vi "TPP-printer-v3.vi"() -> ()   [LabVIEW 2015]
uses:
  <vilib>/DAQmx/write.llb/DAQmx Write (Digital Bool 1Line 1Point).vi
  <vilib>/Utility/file.llb/Read Delimited Spreadsheet (I64).vi
  <vilib>/DAQmx/create/channels.llb/DAQmx Create Channel (DO-Digital Output).vi
  <vilib>/DAQmx/miscellaneous.llb/DAQmx Fill In Error Info.vi
  <vilib>/Platform/NI_3dgraph.lvlib
  Kinesis/Thorlabs.MotionControl.Controls.dll
panel:
  in  "f_objecitve(mm)":dbl=1.8
  in  "f_tubelens(mm)":dbl=200.0
  in  "f_scanlens(mm)":dbl=50.0
  out "%":dbl=1.1971958040155672 format="%#.2g"
  in  "读取点阵文件":path=path "C:/Users/Hongq/Desktop/grating.txt"
  in  "停止":bool
  out "每层耗时/s":dbl format="%#.2g"
  out "每行耗时/s":dbl=0.4888782501220703 format="%#.2g"
  out "每点耗时/ms":dbl=4.009246826171875 format="%#.0g"
  out "当前完成量：":u8(slide)=1 scale=0.0..100.0
  out "耗时/min":dbl=0.11883490880330404 format="%#.2g"
  out "模型XYZ坐标表":dbl[][](array[numeric])
  in  "模型高/um":dbl=1.0
  in  "总体预览":refnum<k7>(container)
  in  "刷新预览":bool
  in  "Z轴驱动序列号":string="27000001"
  in  "KCubeDCServoControl":refnum<k24>(container)
  in  "XY速度(um/s)":dbl
  out "XYZ当前坐标/um":dbl[](array[numeric])=[-0.4166666666666667, -0.1875, 0.0, 7.132113933563232, 7.091063499450684, 0.0] format="%#.2g"
  in  "比例因子(V/°)":dbl=0.5
  in  "AO通道：X前Y后":tag="Dev1/ao0:1"
  out "当前扫描速度(um/s)":dbl
  in  "DO通道：shutter控制":tag="Dev1/port1/line0" caption="线"
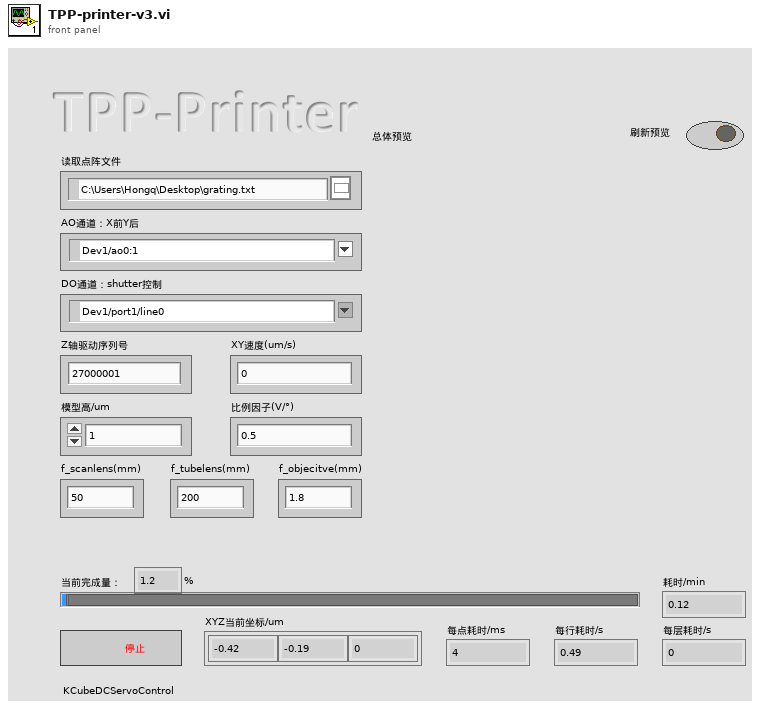
[diagram p1: front panel]
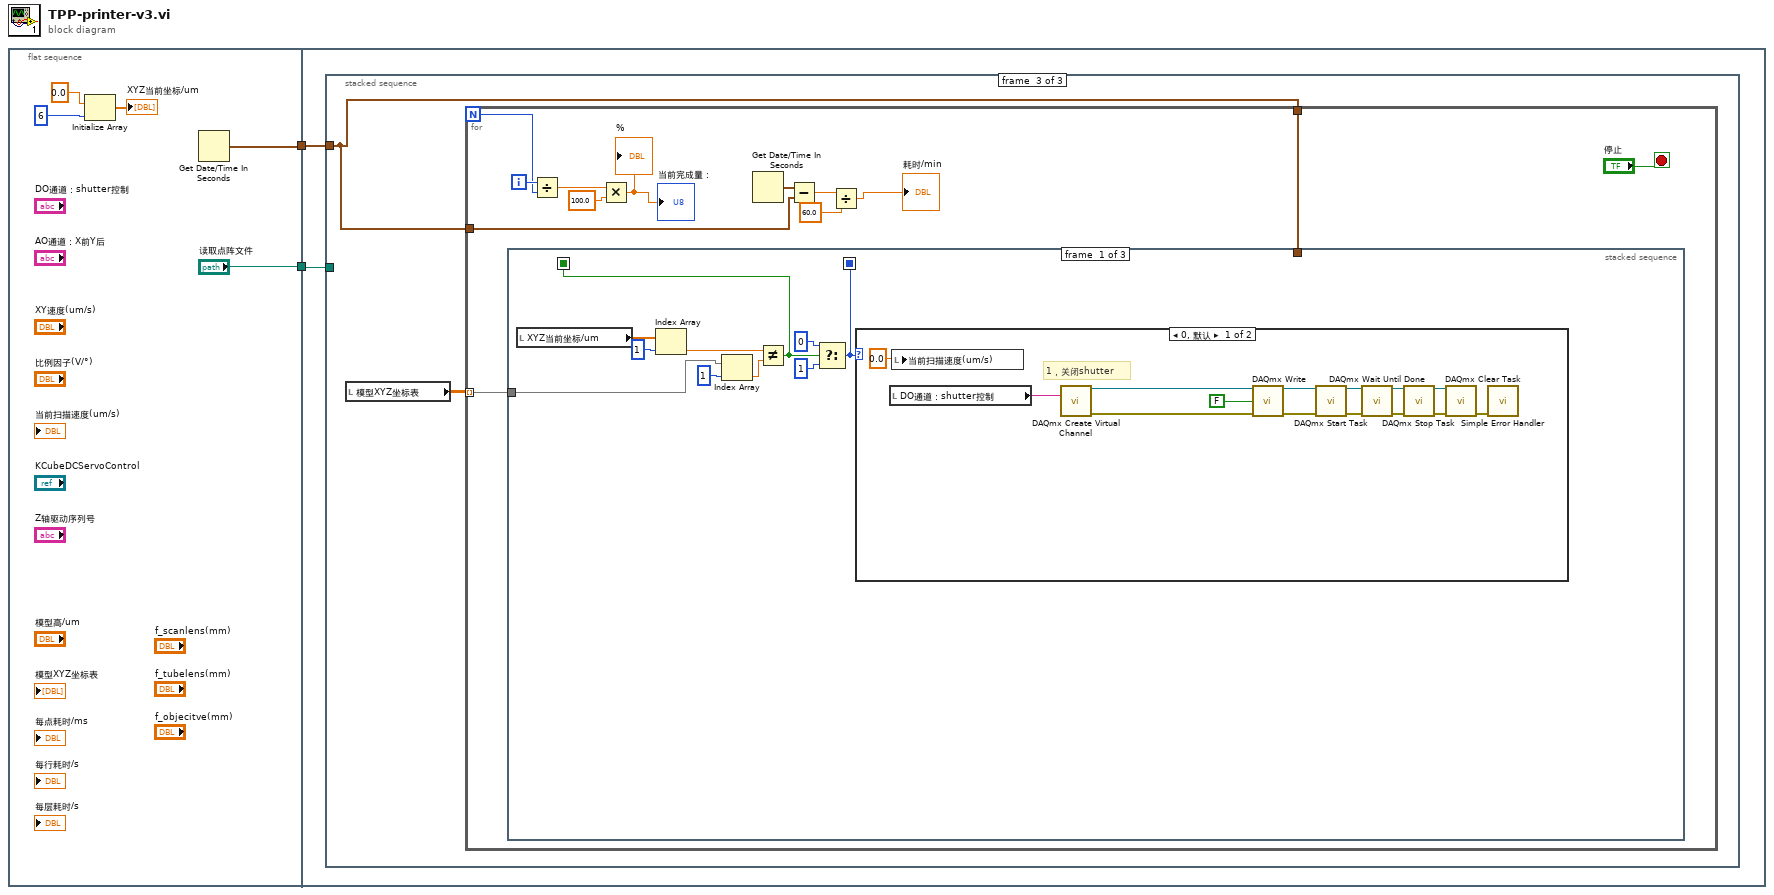
[diagram p0: block diagram]
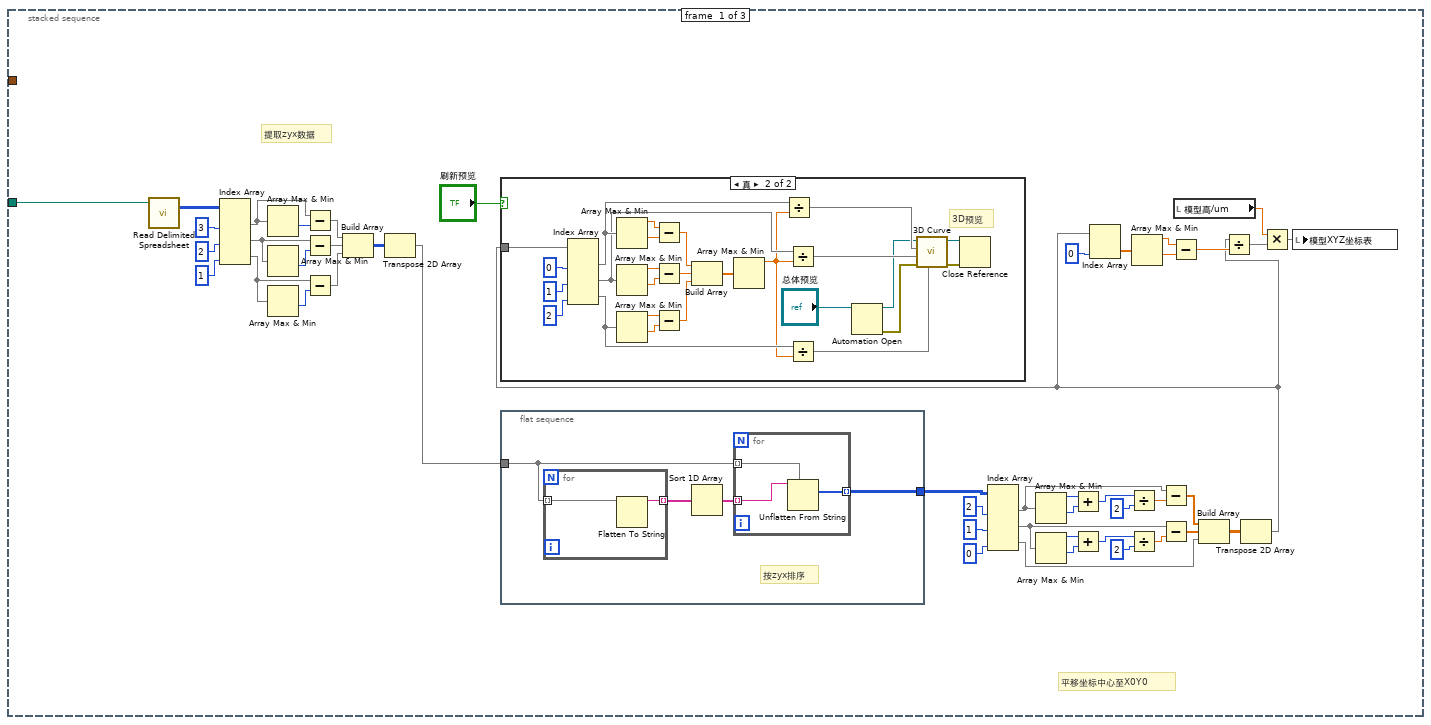
[diagram p2: hidden frame]
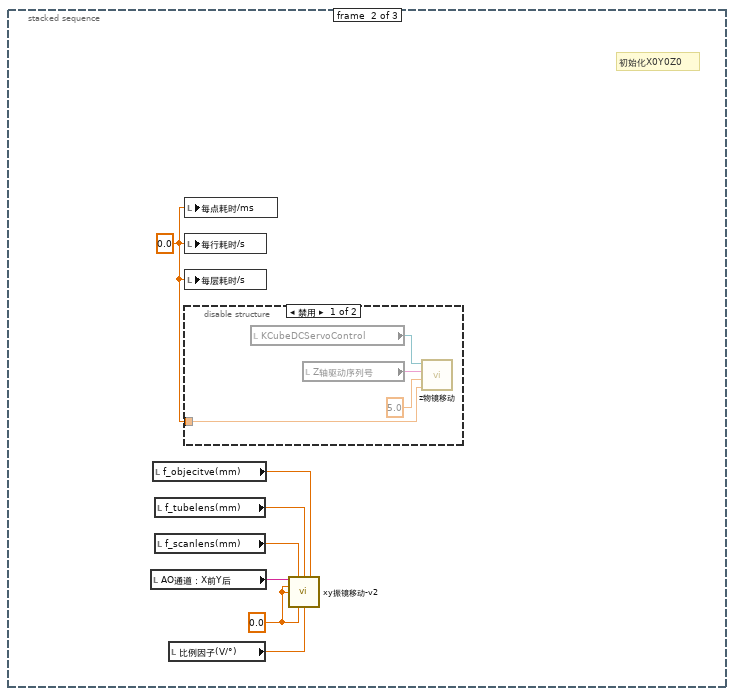
[diagram p4: hidden frame]
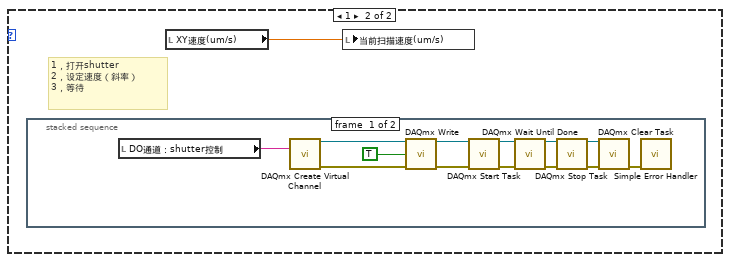
[diagram p6: hidden frame]
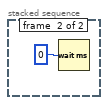
[diagram p7: hidden frame]
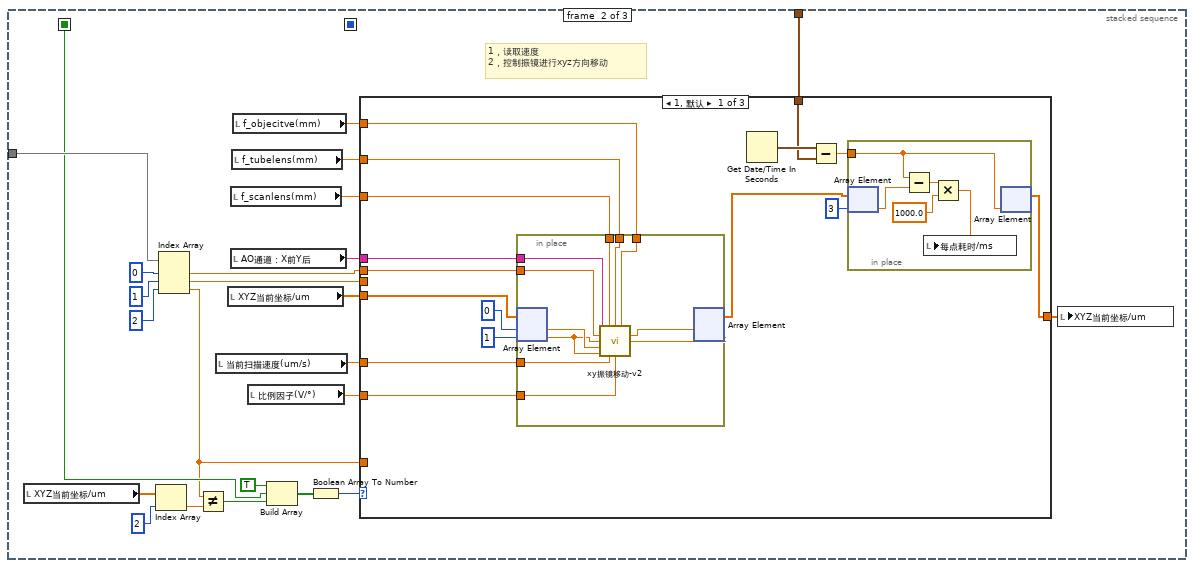
[diagram p8: hidden frame]
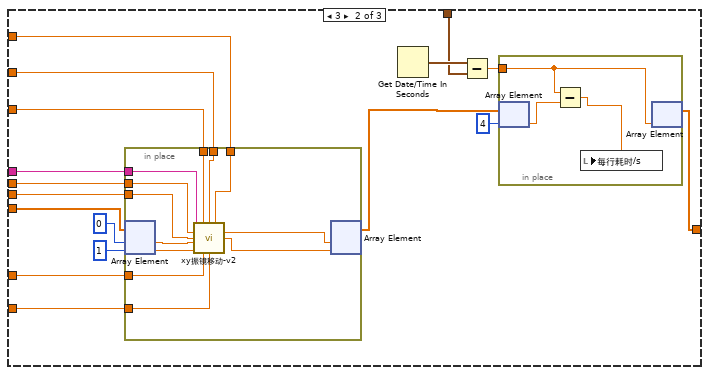
[diagram p9: hidden frame]
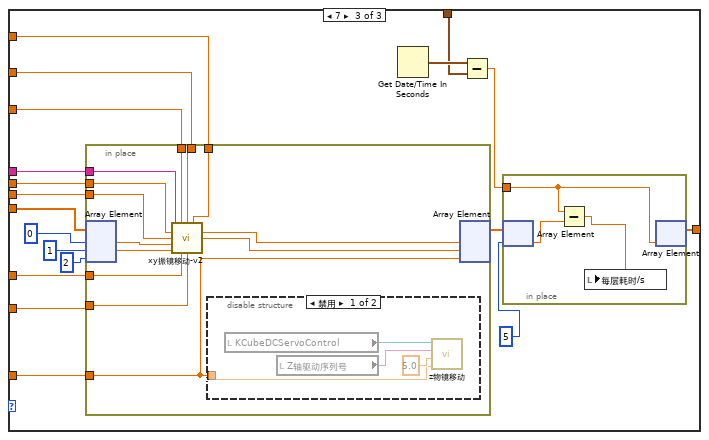
[diagram p10: hidden frame]
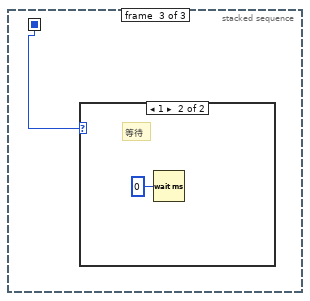
[diagram p12: hidden frame]
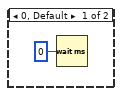
[diagram p13: hidden frame]
diagram:
  n1 = flat-sequence {
    tunnel: [w4] -> w2
    tunnel: ["读取点阵文件"] -> w1
    tunnel: w2 -> [w9]
    tunnel: w1 -> [w8]
    frame #0 {
      n2 = Initialize Array(0.0 ("元素"), 6 ("维数大小")) -> (→"XYZ当前坐标/um":dbl[])
      n3 = Get Date/Time In Seconds() -> (seconds since 1Jan1904=w4:timestamp)
    }
    frame #1 {
      n4 = stacked-sequence {
        tunnel: w9 -> [_ _ w102]
        tunnel: w8 -> [w24 _ _]
        frame #0 {
          # "提取zyx数据"
          # "平移坐标中心至X0Y0"
          n5 = call-poly <vilib>:"Read Delimited Spreadsheet.vi"("file path (dialog if empty)"=w24) -> ("all rows"=w54:i64[][])  [unwired: 9 in, 5 out]
          n6 = Index Array(array=w54, index (col) #1=3 ("禁用的索引 (列)"), index (col) #2=2 ("索引 (列)"), index (col) #3=1 ("索引 (列)")) -> (element #1=w50:i64[], element #2=w52:i64[], element #3=w48:i64[])  [unwired: 3 in]
          n7 = Array Max & Min(array=w50) -> (min value=w42:i64)  [unwired: 3 out]
          n8 = Array Max & Min(array=w52) -> (min value=w40:i64)  [unwired: 3 out]
          n9 = Array Max & Min(array=w48) -> (min value=w41:i64)  [unwired: 3 out]
          n10 = Subtract(x=w50, y=w42) -> (x-y=w51:i64[])
          n11 = Subtract(x=w52, y=w40) -> (x-y=w53:i64[])
          n12 = Subtract(x=w48, y=w41) -> (x-y=w49:i64[])
          n13 = Build Array(w51, w53, w49) -> (w47:i64[][])
          n14 = Transpose 2D Array(2D array=w47) -> (transposed array=w43:i64[][])
          n15 = flat-sequence {
            tunnel: w43 -> [w83]
            tunnel: [w82] -> w27
            frame #0 {
              # "按zyx排序"
              n16 = for {
                tunnel: w83 -> [w90] mode=indexing
                tunnel: [w89] -> w85 mode=indexing
                n17 = Flatten To String(anything=w90) -> (data string=w89:string)  [unwired: 3 in, 2 out]
              }
              n18 = Sort 1D Array(array=w85) -> (sorted array=w84:string[])
              n19 = for {
                tunnel: w84 -> [w88] mode=indexing
                tunnel: w83 -> [w87] mode=indexing
                tunnel: [w86] -> w82 mode=indexing
                n20 = Unflatten From String(type=w87, binary string=w88) -> (value=w86:i64[])  [unwired: 3 in, 2 out]
              }
            }
          }
          n21 = Index Array(array=w27, index (col) #1=2 ("禁用的索引 (列)"), index (col) #2=1 ("索引 (列)"), index (col) #3=0 ("索引 (列)")) -> (element #1=w38:i64[], element #2=w39:i64[], element #3=w12:i64[])  [unwired: 3 in]
          n22 = Array Max & Min(array=w38) -> (max value=w31:i64, min value=w29:i64)  [unwired: 2 out]
          n23 = Array Max & Min(array=w39) -> (max value=w36:i64, min value=w37:i64)  [unwired: 2 out]
          n24 = Add(x=w31, y=w29) -> (x+y=w32:i64)
          n25 = Add(x=w36, y=w37) -> (x+y=w35:i64)
          n26 = Divide(x=w32, y=i64 2) -> (x/y=w28:dbl)
          n27 = Divide(x=w35, y=i64 2) -> (x/y=w33:dbl)
          n28 = Subtract(x=w38, y=w28) -> (x-y=w14:dbl[])
          n29 = Subtract(x=w39, y=w33) -> (x-y=w13:dbl[])
          n30 = local read "模型高/um"() -> (w17:dbl)
          n31 = Build Array(w14, w13, w12) -> (w11:dbl[][])
          n32 = Transpose 2D Array(2D array=w11) -> (transposed array=w10:dbl[][])
          n33 = case shown="真" "刷新预览" {
            tunnel: w10 -> [_ w78]
            frame False {
            }
            frame True {
              # "3D预览"
              n34 = Index Array(array=w78, index (col) #1=0 ("禁用的索引 (列)"), index (col) #2=1 ("索引 (列)"), index (col) #3=2 ("索引 (列)")) -> (element #1=w76:dbl[], element #2=w75:dbl[], element #3=w74:dbl[])  [unwired: 3 in]
              n35 = Array Max & Min(array=w76) -> (max value=w71:dbl, min value=w72:dbl)  [unwired: 2 out]
              n36 = Array Max & Min(array=w75) -> (max value=w69:dbl, min value=w70:dbl)  [unwired: 2 out]
              n37 = Array Max & Min(array=w74) -> (max value=w68:dbl, min value=w67:dbl)  [unwired: 2 out]
              n38 = Subtract(x=w71, y=w72) -> (x-y=w66:dbl)
              n39 = Subtract(x=w69, y=w70) -> (x-y=w65:dbl)
              n40 = Subtract(x=w68, y=w67) -> (x-y=w64:dbl)
              n41 = Build Array(w66, w65, w64) -> (w77:dbl[])
              n42 = Array Max & Min(array=w77) -> (max value=w73:dbl)  [unwired: 3 out]
              n43 = Divide(x=w76, y=w73) -> (x/y=w61:dbl[])
              n44 = Divide(x=w75, y=w73) -> (x/y=w62:dbl[])
              n45 = Divide(x=w74, y=w73) -> (x/y=w63:dbl[])
              n46 = Automation Open(Automation Refnum="总体预览") -> (Automation Refnum=w59:refnum<k7>, error out=w56:errorcluster)  [unwired: 3 in]
              n47 = call <vilib>:"3D Curve.vi"("z vector"=w63, "error in (no error)"=w56, "y vector"=w62, "x vector"=w61, "3D graph"=w59) -> ("error out"=w58:errorcluster, "3D graph out"=w57:refnum<k7>)  [unwired: 5 in]
              n48 = Close Reference(reference=w57, error in (no error)=w58) -> ()  [unwired: 1 out]
            }
          }
          n49 = Index Array(array=w10, index (col)=0 ("禁用的索引 (列)")) -> (element=w21:dbl[])  [unwired: 1 in]
          n50 = Array Max & Min(array=w21) -> (max value=w20:dbl, min value=w19:dbl)  [unwired: 2 out]
          n51 = Subtract(x=w20, y=w19) -> (x-y=w18:dbl)
          n52 = Divide(x=w10, y=w18) -> (x/y=w23:dbl[][])
          n53 = Multiply(x=w17, y=w23) -> (x*y=w16:dbl[][])
          n54 = local write "模型XYZ坐标表"(w16) -> ()
        }
        frame #1 {
          w92 = 0.0 ("每点耗时/ms")
          w91 = 0.0 ("速度(°/s)")
          # "初始化X0Y0Z0"
          n55 = local read "AO通道：X前Y后"() -> (w97:tag)
          n56 = local read "f_objecitve(mm)"() -> (w93:dbl)
          n57 = local read "f_tubelens(mm)"() -> (w94:dbl)
          n58 = local read "f_scanlens(mm)"() -> (w95:dbl)
          n59 = local read "比例因子(V/°)"() -> (w96:dbl)
          n60 = local write "每点耗时/ms"(w92) -> ()
          n61 = local write "每行耗时/s"(w92) -> ()
          n62 = local write "每层耗时/s"(w92) -> ()
          n63 = disable-structure shown="禁用" {
            disable-tunnel: w92 -> [w98 _]
            frame Disabled {
              n64 = local read "KCubeDCServoControl"() -> (w101:refnum<k24>)
              n65 = local read "Z轴驱动序列号"() -> (w100:string)
              n66 = call "z物镜移动.vi"("position"=w98, "maxVelocity"=5.0, "SerialNumber"=w100, "KCubeDCServoControl"=w101) -> ()  [unwired: 5 in, 3 out]
            }
            frame Enabled {
            }
          }
          n67 = call "xy振镜移动-v2.vi"("AO通道：X前Y后"=w97, "f_scanlens(mm)"=w95, "f_tubelens(mm)"=w94, "f_objecitve(mm)"=w93, "x终止位(um)"=w91, "y终止位(um)"=w91, "速度(um/s)"=w91, "比例因子(V/°)"=w96) -> ()  [unwired: 6 in, 2 out]
        }
        frame #2 {
          n68 = local read "模型XYZ坐标表"() -> (w103:dbl[][])
          n69 = for {
            N -> [w114]
            tunnel: w103 -> [w116] mode=indexing
            tunnel: w102 -> [w109]
            tunnel: w102 -> [w104]
            i -> [w115]
            stop <- "停止" stop-if-true
            n70 = stacked-sequence {
              seq-local: [w122 _ _] -> [_ w167 _]
              seq-local: [w117 _ _] -> [_ _ w283]
              tunnel: w116 -> [w125 w178 _]
              tunnel: w104 -> [_ w156 _]
              frame #0 {
                n71 = local read "XYZ当前坐标/um"() -> (w121:dbl[])
                n72 = Index Array(array=w121, index=1 ("索引")) -> (element=w119:dbl)
                n73 = Index Array(array=w125, index=1 ("禁用的索引 (列)")) -> (element=w118:dbl)
                n74 = Not Equal?(x=w119, y=w118) -> (x != y?=w122:bool)
                n75 = Select(t=0, s=w122, f=1) -> (s? t:f=w117:i32)
                n76 = case shown="0, 默认" w117 {
                  frame 0, Default {
                    # "1，关闭shutter"
                    n77 = local read "DO通道：shutter控制"() -> (w128:tag)
                    n78 = local write "当前扫描速度(um/s)"(0.0 ("扫描速度(°/s)")) -> ()
                    n79 = call-poly <vilib>:"DAQmx Create Virtual Channel.vi"("lines"=w128) -> ("task out"=w140:refnum<k21>, "error out"=w139:errorcluster)  [unwired: 13 in]
                    n80 = call-poly <vilib>:"DAQmx Write.vi"("task/channels in"=w140, "data"=FALSE, "error in"=w139) -> ("task out"=w137:refnum<k21>, "error out"=w136:errorcluster)  [unwired: 10 in, 1 out]
                    n81 = call <vilib>:"DAQmx Start Task.vi"("task/channels in"=w137, "error in"=w136) -> ("task out"=w135:refnum<k21>, "error out"=w134:errorcluster)  [unwired: 12 in]
                    n82 = call <vilib>:"DAQmx Wait Until Done.vi"("task/channels in"=w135, "error in"=w134) -> ("task out"=w133:refnum<k21>, "error out"=w132:errorcluster)  [unwired: 12 in]
                    n83 = call <vilib>:"DAQmx Stop Task.vi"("task/channels in"=w133, "error in"=w132) -> ("task out"=w131:refnum<k21>, "error out"=w130:errorcluster)  [unwired: 12 in]
                    n84 = call <vilib>:"DAQmx Clear Task.vi"("task in"=w131, "error in"=w130) -> ("error out"=w129:errorcluster)  [unwired: 13 in]
                    n85 = call <vilib>:"Simple Error Handler.vi"("error in (no error)"=w129) -> ()  [unwired: 4 in, 5 out]
                  }
                  frame 1 {
                    # "1，打开shutter\n2，设定速度（斜率）\n3，等待"
                    n86 = stacked-sequence {
                      frame #0 {
                        n87 = local read "DO通道：shutter控制"() -> (w142:tag)
                        n88 = call-poly <vilib>:"DAQmx Create Virtual Channel.vi"("lines"=w142) -> ("task out"=w154:refnum<k21>, "error out"=w153:errorcluster)  [unwired: 13 in]
                        n89 = call-poly <vilib>:"DAQmx Write.vi"("task/channels in"=w154, "data"=TRUE, "error in"=w153) -> ("task out"=w151:refnum<k21>, "error out"=w150:errorcluster)  [unwired: 10 in, 1 out]
                        n90 = call <vilib>:"DAQmx Start Task.vi"("task/channels in"=w151, "error in"=w150) -> ("task out"=w149:refnum<k21>, "error out"=w148:errorcluster)  [unwired: 12 in]
                        n91 = call <vilib>:"DAQmx Wait Until Done.vi"("task/channels in"=w149, "error in"=w148) -> ("task out"=w147:refnum<k21>, "error out"=w146:errorcluster)  [unwired: 12 in]
                        n92 = call <vilib>:"DAQmx Stop Task.vi"("task/channels in"=w147, "error in"=w146) -> ("task out"=w145:refnum<k21>, "error out"=w144:errorcluster)  [unwired: 12 in]
                        n93 = call <vilib>:"DAQmx Clear Task.vi"("task in"=w145, "error in"=w144) -> ("error out"=w143:errorcluster)  [unwired: 13 in]
                        n94 = call <vilib>:"Simple Error Handler.vi"("error in (no error)"=w143) -> ()  [unwired: 4 in, 5 out]
                      }
                      frame #1 {
                        n95 = Wait (ms)(milliseconds to wait=u32 0 ("等待时间（毫秒）")) -> ()  [unwired: 1 out]
                      }
                    }
                    n96 = local read "XY速度(um/s)"() -> (w141:dbl)
                    n97 = local write "当前扫描速度(um/s)"(w141) -> ()
                  }
                }
              }
              frame #1 {
                # "1，读取速度\n2，控制振镜进行xyz方向移动"
                n98 = local read "XYZ当前坐标/um"() -> (w163:dbl[])
                n99 = Index Array(array=w163, index=2 ("索引")) -> (element=w162:dbl)
                n100 = Index Array(array=w178, index #1=0 ("禁用的索引 (列)"), index #2=1 ("索引"), index #3=2 ("索引")) -> (element #1=w169:dbl, element #2=w166:dbl, element #3=w161:dbl)
                n101 = Not Equal?(x=w161, y=w162) -> (x != y?=w160:bool)
                n102 = local read "当前扫描速度(um/s)"() -> (w175:dbl)
                n103 = local read "XYZ当前坐标/um"() -> (w173:dbl[])
                n104 = local read "f_scanlens(mm)"() -> (w159:dbl)
                n105 = local read "AO通道：X前Y后"() -> (w177:tag)
                n106 = local read "f_tubelens(mm)"() -> (w158:dbl)
                n107 = local read "f_objecitve(mm)"() -> (w157:dbl)
                n108 = local read "比例因子(V/°)"() -> (w176:dbl)
                n109 = Build Array(TRUE ("元素"), w167, w160) -> (w171:bool[])
                n110 = Boolean Array To Number(Boolean array=w171) -> (number=w172:u32)
                n111 = case shown="1, 默认" w172 {
                  tunnel: w177 -> [w190 w223 w259]
                  tunnel: w176 -> [w189 w222 w260]
                  tunnel: w169 -> [w192 w224 w258]
                  tunnel: w173 -> [w195 w225 w257]
                  tunnel: [w180 w212 w244] -> w174
                  tunnel: w175 -> [w191 w226 w256]
                  tunnel: w166 -> [_ w221 w255]
                  tunnel: w161 -> [_ _ w246]
                  tunnel: w159 -> [w188 w220 w254]
                  tunnel: w158 -> [w187 w219 w253]
                  tunnel: w157 -> [w186 w218 w252]
                  tunnel: w156 -> [w184 w214 w248]
                  frame 1, Default {
                    n112 = in-place {
                      in-place-border: w192 -> [w205]
                      in-place-border: w191 -> [w211]
                      in-place-border: w190 -> [w210]
                      in-place-border: w189 -> [w209]
                      in-place-border: w188 -> [w208]
                      in-place-border: w187 -> [w207]
                      in-place-border: w186 -> [w206]
                      n113 = in-place-array #1(w195, 0, 1) -> (w204:dbl, w203:dbl)
                      n114 = call "xy振镜移动-v2.vi"("AO通道：X前Y后"=w210, "f_scanlens(mm)"=w208, "f_tubelens(mm)"=w207, "f_objecitve(mm)"=w206, "x终止位(um)"=w205, "y终止位(um)"=w203, "x初始位(um)"=w204, "y初始位(um)"=w203, "速度(um/s)"=w211, "比例因子(V/°)"=w209) -> ("x终止位(um) 2"=w202:dbl, "y终止位(um) 2"=w201:dbl)  [unwired: 4 in]
                      n115 = in-place-array #1(w202, w201) -> (w181:dbl[])  [unwired: 2 out]
                    }
                    n116 = Get Date/Time In Seconds() -> (seconds since 1Jan1904=w185:timestamp)
                    n117 = Subtract(x=w185, y=w184) -> (x-y=w182:dbl)
                    n118 = in-place {
                      in-place-border: w182 -> [w197]
                      n119 = in-place-array #2(w181, 3) -> (w200:dbl)
                      n120 = Subtract(x=w197, y=w200) -> (x-y=w199:dbl)
                      n121 = Multiply(x=w199, y=1000.0) -> (x*y=w196:dbl)
                      n122 = local write "每点耗时/ms"(w196) -> ()
                      n123 = in-place-array #2(w197) -> (w180:dbl[])  [unwired: 1 out]
                    }
                  }
                  frame 3 {
                    n124 = in-place {
                      in-place-border: w224 -> [w243]
                      in-place-border: w226 -> [w242]
                      in-place-border: w223 -> [w241]
                      in-place-border: w222 -> [w240]
                      in-place-border: w221 -> [w236]
                      in-place-border: w220 -> [w239]
                      in-place-border: w219 -> [w238]
                      in-place-border: w218 -> [w237]
                      n125 = in-place-array #3(w225, 0, 1) -> (w235:dbl, w234:dbl)
                      n126 = call "xy振镜移动-v2.vi"("AO通道：X前Y后"=w241, "f_scanlens(mm)"=w239, "f_tubelens(mm)"=w238, "f_objecitve(mm)"=w237, "x终止位(um)"=w243, "y终止位(um)"=w236, "x初始位(um)"=w235, "y初始位(um)"=w234, "速度(um/s)"=w242, "比例因子(V/°)"=w240) -> ("x终止位(um) 2"=w233:dbl, "y终止位(um) 2"=w232:dbl)  [unwired: 4 in]
                      n127 = in-place-array #3(w233, w232) -> (w213:dbl[])  [unwired: 2 out]
                    }
                    n128 = Get Date/Time In Seconds() -> (seconds since 1Jan1904=w215:timestamp)
                    n129 = Subtract(x=w215, y=w214) -> (x-y=w217:dbl)
                    n130 = in-place {
                      in-place-border: w217 -> [w230]
                      n131 = in-place-array #4(w213, 4) -> (w231:dbl)
                      n132 = Subtract(x=w230, y=w231) -> (x-y=w229:dbl)
                      n133 = local write "每行耗时/s"(w229) -> ()
                      n134 = in-place-array #4(w230) -> (w212:dbl[])  [unwired: 1 out]
                    }
                  }
                  frame 7 {
                    n135 = in-place {
                      in-place-border: w258 -> [w277]
                      in-place-border: w256 -> [w268]
                      in-place-border: w259 -> [w278]
                      in-place-border: w260 -> [w267]
                      in-place-border: w255 -> [w276]
                      in-place-border: w254 -> [w271]
                      in-place-border: w253 -> [w270]
                      in-place-border: w252 -> [w269]
                      in-place-border: w246 -> [w266]
                      n136 = in-place-array #5(w257, 0, 1, 2) -> (w273:dbl, w272:dbl)  [unwired: 1 out]
                      n137 = call "xy振镜移动-v2.vi"("AO通道：X前Y后"=w278, "f_scanlens(mm)"=w271, "f_tubelens(mm)"=w270, "f_objecitve(mm)"=w269, "x终止位(um)"=w277, "y终止位(um)"=w276, "x初始位(um)"=w273, "y初始位(um)"=w272, "速度(um/s)"=w268, "比例因子(V/°)"=w267) -> ("x终止位(um) 2"=w275:dbl, "y终止位(um) 2"=w274:dbl)  [unwired: 4 in]
                      n138 = disable-structure shown="禁用" {
                        disable-tunnel: w266 -> [w279 _]
                        frame Disabled {
                          n139 = local read "KCubeDCServoControl"() -> (w282:refnum<k24>)
                          n140 = local read "Z轴驱动序列号"() -> (w281:string)
                          n141 = call "z物镜移动.vi"("position"=w279, "maxVelocity"=5.0, "SerialNumber"=w281, "KCubeDCServoControl"=w282) -> ()  [unwired: 5 in, 3 out]
                        }
                        frame Enabled {
                        }
                      }
                      n142 = in-place-array #5(w275, w274, w266) -> (w245:dbl[])  [unwired: 3 out]
                    }
                    n143 = Get Date/Time In Seconds() -> (seconds since 1Jan1904=w249:timestamp)
                    n144 = Subtract(x=w249, y=w248) -> (x-y=w251:dbl)
                    n145 = in-place {
                      in-place-border: w251 -> [w264]
                      n146 = in-place-array #6(w245, 5) -> (w265:dbl)
                      n147 = Subtract(x=w264, y=w265) -> (x-y=w263:dbl)
                      n148 = local write "每层耗时/s"(w263) -> ()
                      n149 = in-place-array #6(w264) -> (w244:dbl[])  [unwired: 1 out]
                    }
                  }
                }
                n150 = local write "XYZ当前坐标/um"(w174) -> ()
              }
              frame #2 {
                n151 = case shown="1" w283 {
                  frame 0, Default {
                    n152 = Wait (ms)(milliseconds to wait=u32 0 ("等待时间（毫秒）")) -> ()  [unwired: 1 out]
                  }
                  frame 1 {
                    # "等待"
                    n153 = Wait (ms)(milliseconds to wait=u32 0 ("等待时间（毫秒）")) -> ()  [unwired: 1 out]
                  }
                }
              }
            }
            n154 = Divide(x=w115, y=w114) -> (x/y=w113:dbl)
            n155 = Multiply(x=w113, y=100.0) -> (x*y=→"当前完成量：" →"%":dbl)
            n156 = Get Date/Time In Seconds() -> (seconds since 1Jan1904=w110:timestamp)
            n157 = Subtract(x=w110, y=w109) -> (x-y=w107:dbl)
            n158 = Divide(x=w107, y=60.0) -> (x/y=→"耗时/min":dbl)
          }
        }
      }
    }
  }
